vi "Initialize Front Panel.vi"(8 "error in (no error)":errorcluster, 11 "Car Wash Display ViewManager in":refnum<class "Car Wash Display ViewManager.lvclass">) -> (0 "error out":errorcluster, 3 "Car Wash Display ViewManager out":refnum<class "Car Wash Display ViewManager.lvclass">)   [LabVIEW 2019, in "Car Wash Display ViewManager.lvclass"]
doc: "<License>\nCopyright © 2017 Composed Systems, LLC | All rights reserved\nwww.composed.io\n\nAuthor: Ethan Stern <ethan.stern@composed.io>\n\nThis software is provided \"AS IS\" WITHOUT WARRANTIES, either express or implied, AND IS FOR EDUCATIONAL PURPOSES ONLY.\n</License>"
uses:
  <vilib>/gpm_packages/@cs/Car-wash/Source/Car Wash Display ViewManager/Car Wash Display ViewManager/Car Wash Display ViewManager.lvclass
  <vilib>/gpm_packages/@cs/mva-viewable/Source/IViewManager/IViewManager/IViewManager.lvclass
  <vilib>/gpm_packages/@cs/mva-viewable/Source/IViewable/IViewable Messages/Insert Front Panel Msg/Insert Front Panel Msg.lvclass
  C:/Program Files/National Instruments/LabVIEW 2019/vi.lib/gpm_packages/@cs/mva-viewable/Source/IViewManager/IViewManager/IViewManager.lvclass
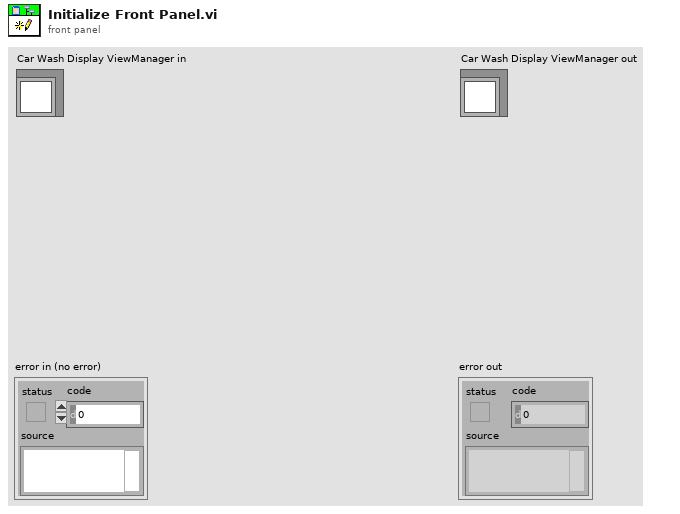
[diagram p1: front panel]
types:
  T1 = typedef "IViewable.lvlib/ProtectedSubpanel.lvclass/Protected Subpanel Reference.ctl" = refnum<data-value>
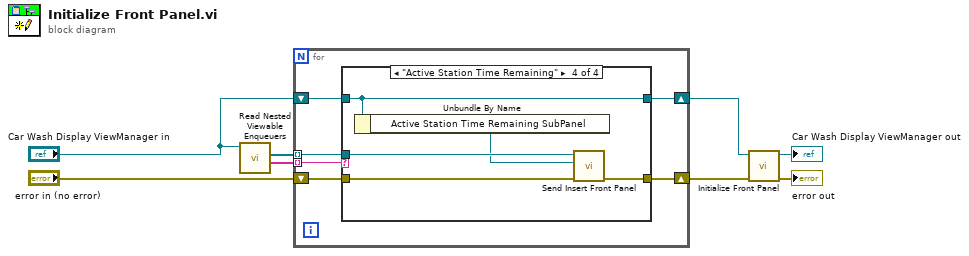
[diagram p0: block diagram]
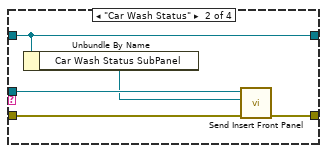
[diagram p3: hidden frame]
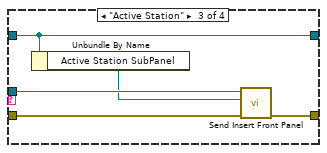
[diagram p4: hidden frame]
diagram:
  n1 = call <vilib>:"Read Nested Viewable Enqueuers.vi"("IViewManager in"="Car Wash Display ViewManager in") -> ("Viewable Names"=w5:string[], "Nested Viewable Enqueuers"=w6:refnum<class "Message Enqueuer.lvclass">[])  [unwired: 9 in]
  n2 = for {
    tunnel: w6 -> [w12] mode=indexing
    tunnel: w5 -> [w9] mode=indexing
    shift-right: [w10] -> w1
    shift-left: "Car Wash Display ViewManager in" -> [w11]
    shift-right: [w13] -> w3
    shift-left: "error in (no error)" -> [w14]
    n3 = case shown="\"Active Station Time Remaining\"" w9 {
      tunnel: w14 -> [w15 w21 w26 w31]
      tunnel: [w15 w20 w25 w30] -> w13
      tunnel: w12 -> [_ w19 w24 w29]
      tunnel: [w16 w18 w23 w28] -> w10
      tunnel: w11 -> [w16 w18 w23 w28]
      frame Default {
      }
      frame "Car Wash Status" {
        n4 = Unbundle By Name(w18) -> ("Car Wash Status SubPanel"=w17:T1)
        n5 = call <vilib>:"Send Insert Front Panel.vi"("error in (no error)"=w21, "Protected Subpanel"=w17, "Message Enqueuer"=w19) -> ("error out"=w20:errorcluster)  [unwired: 7 in, 1 out]
      }
      frame "Active Station" {
        n6 = Unbundle By Name(w23) -> ("Active Station SubPanel"=w22:T1)
        n7 = call <vilib>:"Send Insert Front Panel.vi"("error in (no error)"=w26, "Protected Subpanel"=w22, "Message Enqueuer"=w24) -> ("error out"=w25:errorcluster)  [unwired: 7 in, 1 out]
      }
      frame "Active Station Time Remaining" {
        n8 = Unbundle By Name(w28) -> ("Active Station Time Remaining SubPanel"=w27:T1)
        n9 = call <vilib>:"Send Insert Front Panel.vi"("error in (no error)"=w31, "Protected Subpanel"=w27, "Message Enqueuer"=w29) -> ("error out"=w30:errorcluster)  [unwired: 7 in, 1 out]
      }
    }
  }
  n10 = call-parent "Initialize Front Panel.vi"("error in (no error)"=w3, "IViewable in"=w1) -> ("error out"=→"error out":errorcluster, "IViewable out"=→"Car Wash Display ViewManager out":refnum<class "Car Wash Display ViewManager.lvclass">)  [unwired: 8 in]
